vi "Set LabVIEW Printing Settings.vi"(8 "error in (no error)":errorcluster, 9 "color or monochrome":T2 items=["Unchanged", "Color/grayscale", "Monochrome"], 10 "printing method":T1 items=["Unchanged", "Standard", "PostScript", "Bitmap"], 11 "default printer name":string) -> (0 "error out":errorcluster)   [LabVIEW 2017, in "NI_ReportGenerationCore.lvlib"]
uses:
  <vilib>/Utility/NIReport.llb/NI_ReportGenerationCore.lvlib
  <vilib>/printing/EasyPrintingControls.llb/color_or_monochrome.ctl
  <vilib>/printing/EasyPrintingControls.llb/printing_method.ctl
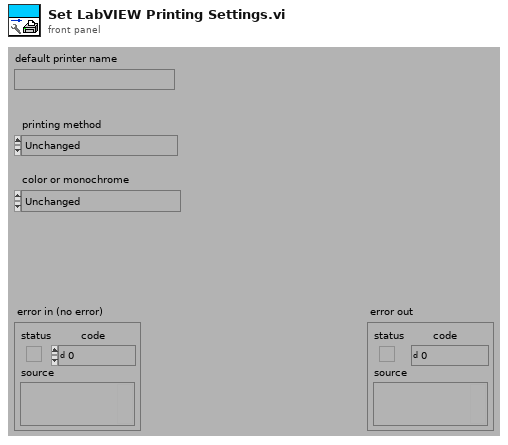
[diagram p1: front panel]
types:
  T1 = typedef "NI_ReportGenerationCore.lvlib/printing_method.ctl" = u16
  T2 = typedef "NI_ReportGenerationCore.lvlib/color_or_monochrome.ctl" = u16
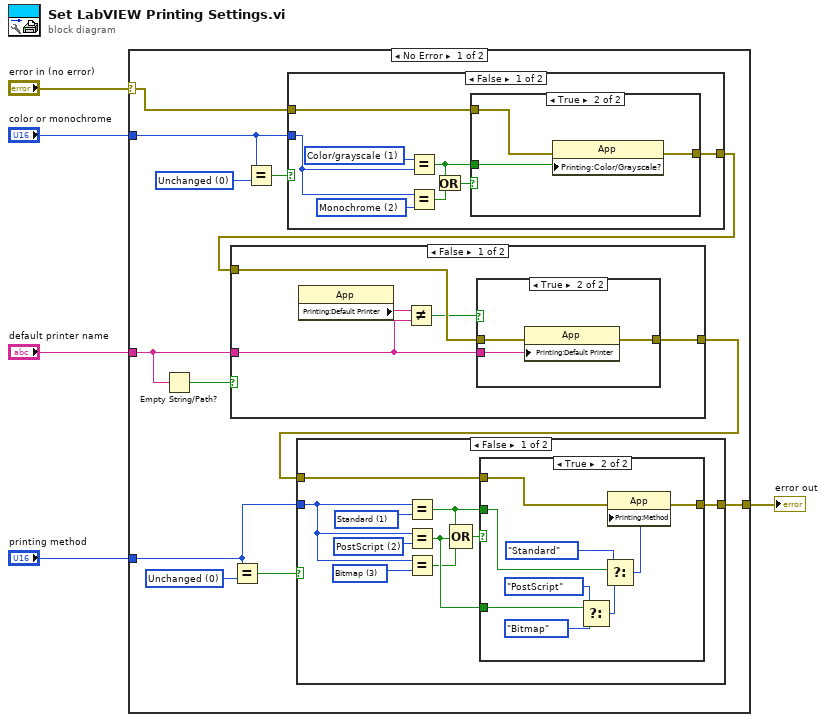
[diagram p0: block diagram]
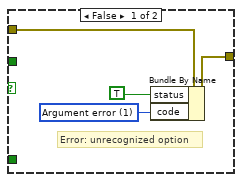
[diagram p4: hidden frame]
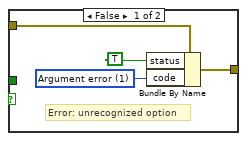
[diagram p6: hidden frame]
diagram:
  n1 = case shown="No Error" "error in (no error)" {
    selector: "error in (no error)" -> [w11 w68]
    tunnel: "default printer name" -> [w17 _]
    tunnel: "color or monochrome" -> [w7 _]
    tunnel: "printing method" -> [w6 _]
    tunnel: [w8 w68] -> w1
    frame No Error {
      w14 = T1 0 items=["Unchanged", "Standard", "PostScript", "Bitmap"] ("printing method")
      w16 = T2 0 items=["Unchanged", "Color/grayscale", "Monochrome"] ("color or monochrome")
      n2 = Empty String/Path?(string/path=w17) -> (empty?=w12:bool)
      n3 = Equal?(x=w6, y=w14) -> (x = y?=w13:bool)
      n4 = Equal?(x=w7, y=w16) -> (x = y?=w15:bool)
      n5 = case shown="False" w15 {
        tunnel: w7 -> [w54 _]
        tunnel: w11 -> [w55 w67]
        tunnel: [w53 w67] -> w10
        frame False {
          w59 = T2 2 items=["Unchanged", "Color/grayscale", "Monochrome"] ("color or monochrome")
          w52 = T2 1 items=["Unchanged", "Color/grayscale", "Monochrome"] ("color or monochrome")
          n6 = Equal?(x=w52, y=w54) -> (x = y?=w57:bool)
          n7 = Equal?(x=w54, y=w59) -> (x = y?=w56:bool)
          n8 = Or(x=w57, y=w56) -> (x .or. y?=w58:bool)
          n9 = case shown="True" w58 {
            tunnel: w55 -> [w63 w66]
            tunnel: [w60 w65] -> w53
            tunnel: w57 -> [_ w64]
            frame False {
              w61 = 1 items=["No error", "Argument error", "Memory is full", "Out of zone", "End of file", "File already open", "Generic file I/O error", "File not found", "File permission error", "Disk is full", "Duplicate path", "Too many files open", "System feature not enabled", "Resource file not found", "Cannot add resource", "Resource not found", "Image not found", "Image memory error", "Pen does not exist", "Config type invalid", "Config token not found", "Config parse error", "Config memory error", "Bad external code format", "Bad external code offset", "External code not present", "Null window", "Destroy window error", "Null menu", "Print aborted", "Bad print record", "Print driver error", "Windows error during printing", "Memory error during printing", "Print dialog error", "Generic print error", "Invalid device refnum", "Device not found", "Device parameter error", "Device unit error", "Cannot open device", "Device call aborted", "Generic error", "Cancelled by user", "Object ID too low", "Object ID too high", "Object not in heap", "Unknown heap", "Unknown object (invalid DefProc)", "Unknown object (DefProc not in table)", "Message out of range", "Invalid (null) method", "Unknown message", "Manager call not supported", "Bad address", "Network operation in progress", "Network operation timed out", "Connection is busy", "Network attribute not supported", "Network error", "Address in use", "System out of memory", "Connection aborted", "Connection refused", "Not connected", "Already connected", "Connection closed", "Initialization error (interapplication manager)", "Bad occurrence", "Wait on unbound occurrence handler", "Occurrence queue overflow", "Datalog type conflict", "Unused", "Unrecognized type (interapplication manager)", "Memory corrupt", "Failed to make temporary DLL", "Old CIN version", "Drag socket not found", "Failed to load drop-object", "Failed to register OLE object", "Failed to release OLE object", "Format specifier type mismatch", "Unknown format specifier", "Too few format specifiers", "Too many format specifiers", "Scan failed", "Newer CIN version", "Error converting to variant", "Runtime menu error", "Password tampered", "Variant attribute not found", "Incompatible variant data type", "Event data is not available", "Event Store is not present", "Occurrence is not found", "Event Queue is not created", "Event info is not available", "Refnum passed is NULL", "Error retrieving Class GUID", "Error retrieving CoClass GUID", "Error retrieving TypeLib GUID.", "Bad built application magic bytes.", "Specific driver is different from the specific driver associated with the Logical Name.", "There is no session opened to the class driver.", "Max Error", "MAX - Error with config objects", "MAX - Error loading configuration", "MAX - Group not supported"]
              # "Error: unrecognized option"
              n10 = Bundle By Name(cluster=w63, "status"=TRUE, "code"=w61) -> (w60:errorcluster)
            }
            frame True {
              n11 = property class="App"(error in=w66, "Printing:Color/Grayscale?"=w64) -> (error out=w65:errorcluster)  [unwired: 1 in, 1 out]
            }
          }
        }
        frame True {
          # "Do not change this setting"
        }
      }
      n12 = case shown="False" w12 {
        tunnel: w17 -> [w19 _]
        tunnel: w10 -> [w22 w27]
        tunnel: [w21 w27] -> w9
        frame False {
          n13 = property class="App"() -> ("Printing:Default Printer"=w20:string)  [unwired: 2 in, 2 out]
          n14 = Not Equal?(x=w20, y=w19) -> (x != y?=w18:bool)
          n15 = case shown="True" w18 {
            tunnel: w22 -> [w23 w26]
            tunnel: [w23 w25] -> w21
            tunnel: w19 -> [_ w24]
            frame False {
            }
            frame True {
              n16 = property class="App"(error in=w26, "Printing:Default Printer"=w24) -> (error out=w25:errorcluster)  [unwired: 1 in, 1 out]
            }
          }
        }
        frame True {
          # "Do not change this setting"
        }
      }
      n17 = case shown="False" w13 {
        tunnel: w6 -> [w30 _]
        tunnel: w9 -> [w37 w51]
        tunnel: [w36 w51] -> w8
        frame False {
          w33 = T1 3 items=["Unchanged", "Standard", "PostScript", "Bitmap"] ("printing method")
          w34 = T1 2 items=["Unchanged", "Standard", "PostScript", "Bitmap"] ("printing method")
          w35 = T1 1 items=["Unchanged", "Standard", "PostScript", "Bitmap"] ("printing method")
          n18 = Equal?(x=w30, y=w35) -> (x = y?=w28:bool)
          n19 = Equal?(x=w30, y=w34) -> (x = y?=w32:bool)
          n20 = Equal?(x=w30, y=w33) -> (x = y?=w29:bool)
          n21 = Compound Arithmetic op=OR(w28, w32, w29) -> (w31:bool)
          n22 = case shown="True" w31 {
            tunnel: w37 -> [w41 w50]
            tunnel: [w38 w49] -> w36
            tunnel: w28 -> [_ w48]
            tunnel: w32 -> [_ w47]
            frame False {
              w39 = 1 items=["No error", "Argument error", "Memory is full", "Out of zone", "End of file", "File already open", "Generic file I/O error", "File not found", "File permission error", "Disk is full", "Duplicate path", "Too many files open", "System feature not enabled", "Resource file not found", "Cannot add resource", "Resource not found", "Image not found", "Image memory error", "Pen does not exist", "Config type invalid", "Config token not found", "Config parse error", "Config memory error", "Bad external code format", "Bad external code offset", "External code not present", "Null window", "Destroy window error", "Null menu", "Print aborted", "Bad print record", "Print driver error", "Windows error during printing", "Memory error during printing", "Print dialog error", "Generic print error", "Invalid device refnum", "Device not found", "Device parameter error", "Device unit error", "Cannot open device", "Device call aborted", "Generic error", "Cancelled by user", "Object ID too low", "Object ID too high", "Object not in heap", "Unknown heap", "Unknown object (invalid DefProc)", "Unknown object (DefProc not in table)", "Message out of range", "Invalid (null) method", "Unknown message", "Manager call not supported", "Bad address", "Network operation in progress", "Network operation timed out", "Connection is busy", "Network attribute not supported", "Network error", "Address in use", "System out of memory", "Connection aborted", "Connection refused", "Not connected", "Already connected", "Connection closed", "Initialization error (interapplication manager)", "Bad occurrence", "Wait on unbound occurrence handler", "Occurrence queue overflow", "Datalog type conflict", "Unused", "Unrecognized type (interapplication manager)", "Memory corrupt", "Failed to make temporary DLL", "Old CIN version", "Drag socket not found", "Failed to load drop-object", "Failed to register OLE object", "Failed to release OLE object", "Format specifier type mismatch", "Unknown format specifier", "Too few format specifiers", "Too many format specifiers", "Scan failed", "Newer CIN version", "Error converting to variant", "Runtime menu error", "Password tampered", "Variant attribute not found", "Incompatible variant data type", "Event data is not available", "Event Store is not present", "Occurrence is not found", "Event Queue is not created", "Event info is not available", "Refnum passed is NULL", "Error retrieving Class GUID", "Error retrieving CoClass GUID", "Error retrieving TypeLib GUID.", "Bad built application magic bytes.", "Specific driver is different from the specific driver associated with the Logical Name.", "There is no session opened to the class driver.", "Max Error", "MAX - Error with config objects", "MAX - Error loading configuration", "MAX - Group not supported"]
              # "Error: unrecognized option"
              n23 = Bundle By Name(cluster=w41, "status"=TRUE, "code"=w39) -> (w38:errorcluster)
            }
            frame True {
              n24 = Select(t=enum32{"Standard", "PostScript", "Bitmap"}."PostScript" ("Printing:Print Method"), s=w47, f=enum32{"Standard", "PostScript", "Bitmap"}."Bitmap" ("Printing:Print Method")) -> (s? t:f=w46:enum32{"Standard", "PostScript", "Bitmap"})
              n25 = Select(t=enum32{"Standard", "PostScript", "Bitmap"}."Standard" ("Printing:Print Method"), s=w48, f=w46) -> (s? t:f=w45:enum32{"Standard", "PostScript", "Bitmap"})
              n26 = property class="App"(error in=w50, "Printing:Method"=w45) -> (error out=w49:errorcluster)  [unwired: 1 in, 1 out]
            }
          }
        }
        frame True {
          # "Do not change this setting"
        }
      }
    }
    frame Error {
    }
  }
  "error out" <- w1
